vi "api_mqttInit.vi"(0 "client":string="LabVIEW_MQTT_Client", 5 "broker":T4={"address"="localhost", "port"=1883, "connTimeout"=2000, "writeTimeout"=2000, "readTimeout"=2000, "subTimeout"=30000}, 7 "connFlags":T3={"reserved"=FALSE, "clean session"=TRUE, "will flag"=TRUE, "willQOS"=enum."At most once", "will retain"=FALSE, "password"=FALSE, "user name"=FALSE}, 9 "User Info":T2={"User Name"="User", "Password"="password"}, 11 "error in (no error)":errorcluster, 12 "Will Info":T1={"Will message"="Last Will", "Will Topic"="Will Topic"}) -> (15 "error out":errorcluster)   [LabVIEW 2017, in "mqtt.lvclass"]
uses:
  mqtt.lvclass
  mqttTypedef/mqttBroker.ctl
  mqttTypedef/mqttConnectionFlags.ctl
  mqttTypedef/mqttWillInformation.ctl
  mqttTypedef/mqttUserInformation.ctl
  mqttConfigFunction.ctl
  mqtt.lvclass/mqtt.ctl
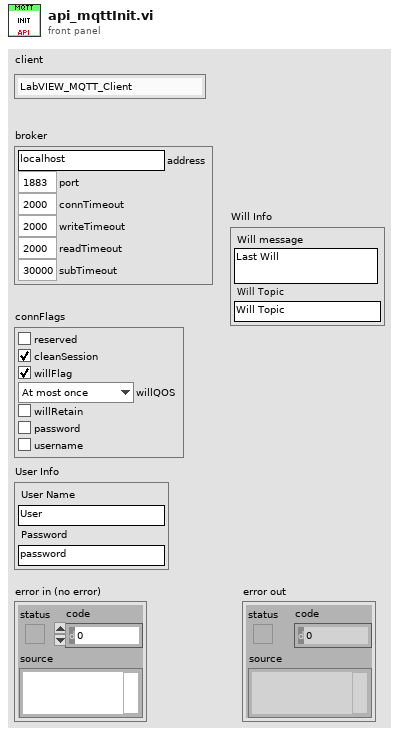
[diagram p1: front panel]
types:
  T1 = typedef "mqttUserInformation.ctl" = cluster{"Will message":string, "Will Topic":string}
  T2 = typedef "mqttWillInformation.ctl" = cluster{"User Name":string, "Password":string}
  T3 = typedef "mqttConnectionFlags.ctl" = cluster{"reserved":bool, "clean session":bool, "will flag":bool, "willQOS":enum8{"At most once", "At least once", "Exactly once", "Reserved"}, "will retain":bool, "password":bool, "user name":bool}
  T4 = typedef "mqttBroker.ctl" = cluster{"address":string, "port":u16, "connTimeout":i32, "writeTimeout":i32, "readTimeout":i32, "subTimeout":i32}
  T5 = typedef "mqtt.lvclass/mqttConfigFunction.ctl" = enum16{"init", "deinit", "set", "get"}
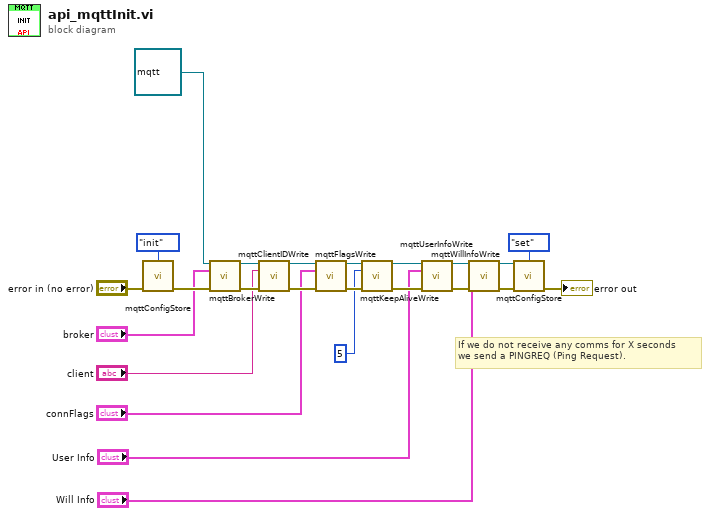
[diagram p0: block diagram]
diagram:
  # "If we do not receive any comms for X seconds\nwe send a PINGREQ (Ping Request)."
  n1 = call "mqttConfigStore.vi"("function"=mqttConfigFunction."init", "error in (no error)"="error in (no error)") -> ("error out"=w13:errorcluster)  [unwired: 12 in, 1 out]
  n2 = call "mqttBrokerWrite.vi"("mqtt in"=refnum<class "mqtt.lvclass"> refnum ("mqtt.lvclass"), "broker"="broker", "error in (no error)"=w13) -> ("mqtt out"=w24:refnum<class "mqtt.lvclass">, "error out"=w23:errorcluster)  [unwired: 11 in]
  n3 = call "mqttClientIDWrite.vi"("mqtt in"=w24, "clientID"="client", "error in (no error)"=w23) -> ("mqtt out"=w19:refnum<class "mqtt.lvclass">, "error out"=w18:errorcluster)  [unwired: 11 in]
  n4 = call "mqttFlagsWrite.vi"("mqtt in"=w19, "connFlags"="connFlags", "error in (no error)"=w18) -> ("mqtt out"=w21:refnum<class "mqtt.lvclass">, "error out"=w20:errorcluster)  [unwired: 11 in]
  n5 = call "mqttKeepAliveWrite.vi"("mqtt in"=w21, "keepAlive(sec)"=u16 5, "error in (no error)"=w20) -> ("mqtt out"=w8:refnum<class "mqtt.lvclass">, "error out"=w7:errorcluster)  [unwired: 11 in]
  n6 = call "mqttUserInfoWrite.vi"("mqtt in"=w8, "User Info"="User Info", "error in (no error)"=w7) -> ("mqtt out"=w5:refnum<class "mqtt.lvclass">, "error out"=w4:errorcluster)  [unwired: 11 in]
  n7 = call "mqttWillInfoWrite.vi"("mqtt in"=w5, "Will Info"="Will Info", "error in (no error)"=w4) -> ("mqtt out"=w3:refnum<class "mqtt.lvclass">, "error out"=w2:errorcluster)  [unwired: 11 in]
  n8 = call "mqttConfigStore.vi"("mqtt.lvclass in"=w3, "function"=mqttConfigFunction."set", "error in (no error)"=w2) -> ("error out"=→"error out":errorcluster)  [unwired: 11 in, 1 out]
